vi "Ramp Status.vi"(8 "error in (no error)":errorcluster, 10 "Loop (1:Loop 1)":u16(ring)=1 items=["Loop 1"=1, "Loop 2"=2], 11 "VISA resource name":refnum<visa-resource-name>) -> (0 "error out":errorcluster, 1 "Ramp Active":bool, 2 "Ramp On":bool, 3 "VISA resource name out":refnum<visa-resource-name>, 5 "Rate Value (0.0)":dbl format="%.1f")   [LabVIEW 2019, in "Lake Shore 325.lvlib"]
doc: "This VI returns the status of the setpoint ramp function. The Model 325 generates a smooth setpoint ramp when the setpoint units are expressed in temperature. Once the ramp feature is turned on, its action is initiated by a setpoint change. When a new setpoint is entered, the instrument changes the setpoint temperature from the old value to the new value at the ramp rate."
uses:
  Lake Shore 325.lvlib
  Instance           1 19Saved   Ramp Status .vi
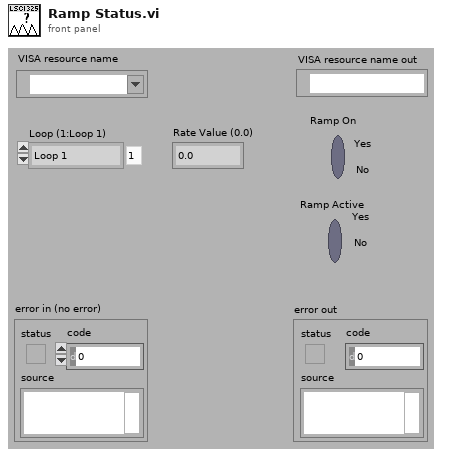
[diagram p1: front panel]
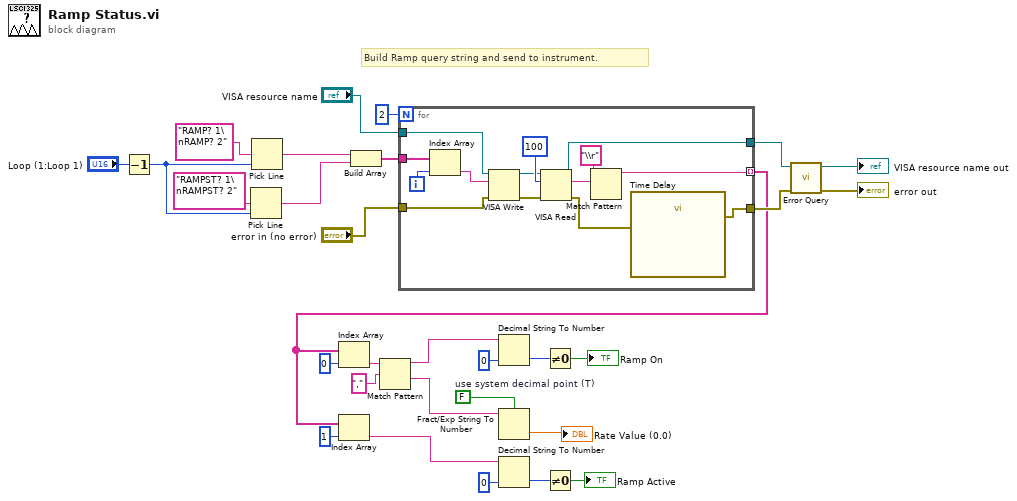
[diagram p0: block diagram]
diagram:
  w28 = FALSE  # use system decimal point (T)
  # "Build Ramp query string and send to instrument."
  n1 = Decrement(x="Loop (1:Loop 1)") -> (x-1=w19:u16)
  n2 = Pick Line(multi-line string="RAMPST? 1\nRAMPST? 2", line index=w19) -> (output string=w16:string)  [unwired: 1 in]
  n3 = Pick Line(multi-line string="RAMP? 1\nRAMP? 2", line index=w19) -> (output string=w17:string)  [unwired: 1 in]
  n4 = Build Array(w17, w16) -> (w18:string[])
  n5 = for {
    N: 2 -> [_]
    tunnel: [w38] -> w26
    tunnel: [w31] -> w25
    tunnel: "VISA resource name" -> [w37]
    tunnel: "error in (no error)" -> [w36]
    tunnel: w18 -> [w35]
    tunnel: [w34] -> w6 mode=indexing
    i -> [w39]
    n6 = Index Array(array=w35, index=w39) -> (element=w33:string)
    n7 = VISA Write(VISA resource name=w37, write buffer=w33, error in (no error)=w36) -> (VISA resource name out=w41:refnum<visa-resource-name>, error out=w40:errorcluster)  [unwired: 1 out]
    n8 = VISA Read(VISA resource name=w41, byte count=100, error in (no error)=w40) -> (VISA resource name out=w38:refnum<visa-resource-name>, read buffer=w43:string, error out=w32:errorcluster)  [unwired: 1 out]
    n9 = Match Pattern(string=w43, regular expression="\\r") -> (before substring=w34:string)  [unwired: 1 in, 3 out]
    n10 = call "Time Delay"("error in (no error)"=w32) -> ("error out"=w31:errorcluster)  [unwired: 10 in]
  }
  n11 = Index Array(array=w6, index=0) -> (element=w7:string)
  n12 = Index Array(array=w6, index=1) -> (element=w2:string)
  n13 = Match Pattern(string=w7, regular expression=",") -> (before substring=w4:string, after substring=w3:string)  [unwired: 1 in, 2 out]
  n14 = Decimal String To Number(string=w4, default (0L)=u16 0) -> (number=w14:u16)  [unwired: 1 in, 1 out]
  n15 = Fract/Exp String To Number(use system decimal point (T)=w28, string=w3) -> (number=→"Rate Value (0.0)":dbl)  [unwired: 2 in, 1 out]
  n16 = Decimal String To Number(string=w2, default (0L)=u16 0) -> (number=w12:u16)  [unwired: 1 in, 1 out]
  n17 = Not Equal To 0?(x=w14) -> (x != 0?=→"Ramp On":bool)
  n18 = Not Equal To 0?(x=w12) -> (x != 0?=→"Ramp Active":bool)
  n19 = call "Error Query.vi"("error in (no error)"=w25, "VISA resource name"=w26) -> ("error out"=→"error out":errorcluster, "VISA resource name out"=→"VISA resource name out":refnum<visa-resource-name>)  [unwired: 7 in, 1 out]
